vi "Launch UI.vi"(6 "Auto-open":bool, 8 "error in (no error)":errorcluster, 11 "Mag Lab Measure Base in":refnum<class "Mag Lab Measure Base.lvclass">) -> (0 "error out":errorcluster, 3 "Mag Lab Measure Base out":refnum<class "Mag Lab Measure Base.lvclass">)   [LabVIEW 2015, in "Mag Lab Measure Base.lvclass"]
uses:
  Mag Lab Measure Base.lvclass
  Mag Lab Measure Base.lvclass/Mag Lab Measure Base.ctl
  <vilib>/ActorFramework/Message Enqueuer/Message Enqueuer.lvclass/Message Enqueuer.ctl
  Mag Lab Root/Mag Lab Root.lvclass/Mag Lab Root.ctl
  Mag Lab Measure Interface/Mag Lab Measure UI.lvclass/Mag Lab Measure UI.ctl
  Mag Lab Root/Read Name.vi
  Mag Lab Root/Write Name.vi
  Mag Lab Measure Interface/Write Auto-open.vi
  <vilib>/ActorFramework/Message Enqueuer/Enqueue.vi
  <vilib>/ActorFramework/Message Priority Queue/Priority Enqueue.vi
  <vilib>/ActorFramework/Message Enqueuer/Message Enqueuer.lvclass
  <vilib>/ActorFramework/Stop Msg/Stop Msg.lvclass
  Mag Lab Properties/Mag Lab Parameters.lvclass
  Mag Lab Measure Interface/Mag Lab Measure UI.lvclass
  <vilib>/ActorFramework/Actor/Actor.lvclass
  Mag Lab Error Handler/Mag Lab Error Handler.lvclass
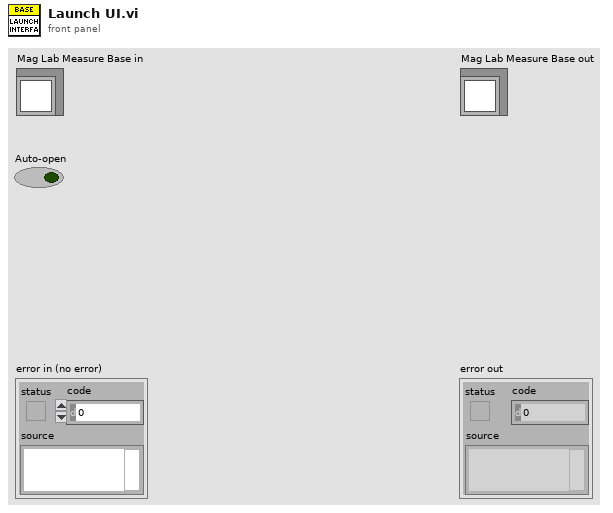
[diagram p1: front panel]
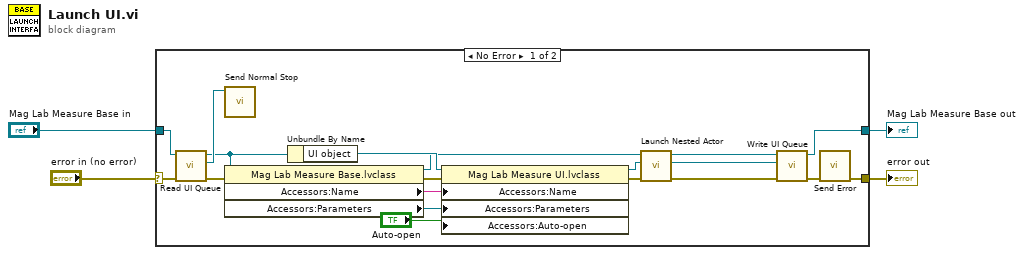
[diagram p0: block diagram]
diagram:
  n1 = case shown="No Error" "error in (no error)" {
    selector: "error in (no error)" -> [w20 w25]
    tunnel: [w18 w25] -> w3
    tunnel: [w16 w24] -> w1
    tunnel: "Mag Lab Measure Base in" -> [w22 w24]
    frame No Error {
      n2 = call "Read UI Queue.vi"("error in (no error)"=w20, "Mag Lab Measure Base in"=w22) -> ("error out"=w7:errorcluster, "Actor Framework.lvlib:Message Enqueuer"=w21:refnum<class "Message Enqueuer.lvclass">, "Mag Lab Measure Base out"=w14:refnum<class "Mag Lab Measure Base.lvclass">)  [unwired: 7 in]
      n3 = call <vilib>:"Send Normal Stop.vi"("Message Enqueuer"=w21) -> ()  [unwired: 10 in, 1 out]
      n4 = property class="Mag Lab Measure Base.lvclass"(reference=w14, error in=w7) -> (reference out=w8:refnum<class "Mag Lab Measure Base.lvclass">, error out=w10:errorcluster, "Accessors:Name"=w12:string, "Accessors:Parameters"=w11:refnum<class "Mag Lab Parameters.lvclass">)
      n5 = Unbundle By Name(w14) -> ("UI object"=w13:refnum<class "Mag Lab Measure UI.lvclass">)
      n6 = property class="Mag Lab Measure UI.lvclass"(reference=w13, error in=w10, "Accessors:Name"=w12, "Accessors:Parameters"=w11, "Accessors:Auto-open"="Auto-open") -> (reference out=w9:refnum<class "Mag Lab Measure UI.lvclass">, error out=w6:errorcluster)
      n7 = call <vilib>:"Launch Nested Actor.vi"("error in (no error)"=w6, "Nested Actor"=w9, "Caller Actor in"=w8) -> ("error out"=w19:errorcluster, "Nested Actor's Enqueuer"=w23:refnum<class "Message Enqueuer.lvclass">, "Caller Actor out"=w17:refnum<class "Mag Lab Measure Base.lvclass">)  [unwired: 6 in]
      n8 = call "Write UI Queue.vi"("error in (no error)"=w19, "Actor Framework.lvlib:Message Enqueuer"=w23, "Mag Lab Measure Base in"=w17) -> ("error out"=w15:errorcluster, "Mag Lab Measure Base out"=w16:refnum<class "Mag Lab Measure Base.lvclass">)  [unwired: 7 in]
      n9 = call "Send Error.vi"("error in (no error)"=w15) -> ("error out"=w18:errorcluster)  [unwired: 9 in, 1 out]
    }
    frame Error {
    }
  }
  "error out" <- w3
  "Mag Lab Measure Base out" <- w1
